vi "LVRT Serial Close.vi"(8 "error out":errorcluster, 11 "FPGA Main Ref":refnum<k20>) -> (0 "error out":errorcluster)   [LabVIEW 2014]
uses:
  <vilib>/Utility/error.llb/Error Cluster From Error Code.vi
  <vilib>/rvi/errors/niLvFpgaAdjustHostInterfaceError.vi
  <vilib>/FPGAPlugInAG/myRIO-1900/niLvFpga_Close_myRIO-1900.vi
  <vilib>/rvi/interface/nirviReadWriteControl/nirviReadWriteControl.xnode
  FPGA Bitfiles/mySynth_FPGATarget_FPGAMain_WASpsvx+XwM.lvbitx
  FPGA Main.vi
  <vilib>/rvi/interface/nirviCloseFPGA/nirviCloseFPGA.xnode
  NiFpgaLv.dll
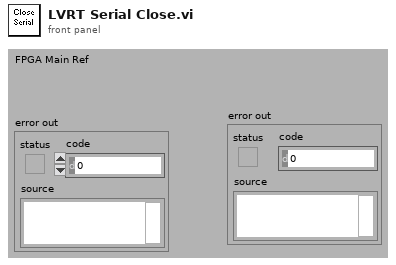
[diagram p1: front panel]
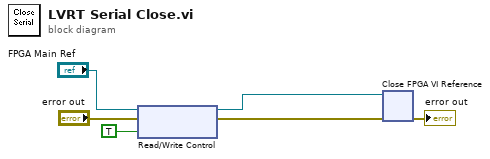
[diagram p0: block diagram]
diagram:
  n1 = xnode "Read/Write Control"("FPGA VI Reference In"="FPGA Main Ref", "error in"="error out", "FPGA STOP"=TRUE ("stop")) -> ("FPGA VI Reference Out"=w2:refnum<k20>, "error out"=w1:errorcluster)
  n2 = xnode "Close FPGA VI Reference"("FPGA VI Reference In"=w2, "error in"=w1) -> ("error out"=→"error out":errorcluster)
